vi "PipeJetComm.vi"(10 "Stroke Velocity (um/ms)":dbl, 11 "Stroke (um)":dbl) -> (2 "Portname":string, 3 ".NET Refnum out":refnum<k24>)   [LabVIEW 2021]
uses:
  C:/Users/csaerome/Documents/PipeJet/PipeJet/Software/bfx_piezo_r13.dll
  Documents/PipeJet/PipeJet/Software/bfx_piezo_r13.dll
panel:
  # "Range of Stroke is 10 - 35 um"
  # "Water-based solvent 60-100;\nViscous solution > 150."
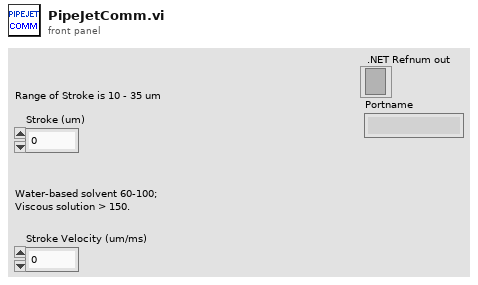
[diagram p1: front panel]
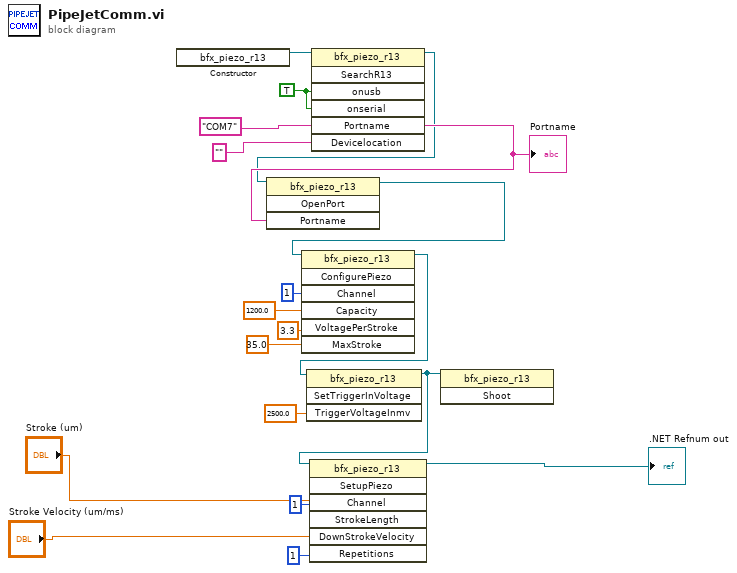
[diagram p0: block diagram]
diagram:
  w15 = TRUE ("onusb")
  n1 = constructor class="bfx_piezo_r13"() -> (reference out=w11:refnum<k24>)  [unwired: 3 in, 2 out]
  n2 = invoke class="bfx_piezo_r13" method="SearchR13"(reference=w11, "onusb"=w15, "onserial"=w15, "Portname"="COM7", "Devicelocation"="") -> (reference out=w10:refnum<k24>, "Portname"=w12:string)  [unwired: 2 in, 5 out]
  "Portname" <- w12
  n3 = invoke class="bfx_piezo_r13" method="OpenPort"(reference=w10, "Portname"=w12) -> (reference out=w5:refnum<k24>)  [unwired: 2 in, 3 out]
  n4 = invoke class="bfx_piezo_r13" method="ConfigurePiezo"(reference=w5, "Channel"=1, "Capacity"=1200.0, "VoltagePerStroke"=3.3, "MaxStroke"=35.0) -> (reference out=w4:refnum<k24>)  [unwired: 2 in, 6 out]
  n5 = invoke class="bfx_piezo_r13" method="SetTriggerInVoltage"(reference=w4, "TriggerVoltageInmv"=2500.0) -> (reference out=w1:refnum<k24>)  [unwired: 2 in, 3 out]
  n6 = invoke class="bfx_piezo_r13" method="SetupPiezo"(reference=w1, "Channel"=1, "StrokeLength"="Stroke (um)", "DownStrokeVelocity"="Stroke Velocity (um/ms)", "Repetitions"=1) -> (reference out=→".NET Refnum out":refnum<k24>)  [unwired: 2 in, 6 out]
  n7 = invoke class="bfx_piezo_r13" method="Shoot"(reference=w1) -> ()  [unwired: 2 in, 3 out]
